vi "FILE Open.vi"(5 "Pattern":string, 6 "Default Name":string, 7 "Dialog Prompt":string, 8 "Error In (no error)":errorcluster, 10 "Start path":path=path "", 11 "File Path (\" \")":path) -> (0 "Error Out":errorcluster, 1 "Size (bytes)":i32, 2 "Dup File Path":path, 3 "Refnum":refnum<file>, 4 "Last Mod":u32)   [LabVIEW 2011]
doc: "This VI opens a file at the file path specified and returns the file's size, mod date, refnum, and dir/file info. If the File Path is empty then a file dialog will appear according to the dialog input parameters given, and the file chosen will be opened. If the file dialog is canceled then execution will continue with no errors.\n\nThis vi was created by David Gianetto, contact me with any problems, questions, etc."
uses:
  Type Defs/FILE Open Mode Enum.ctl
panel:
  out "Directory":bool
  in  "Open Mode (0)":T1
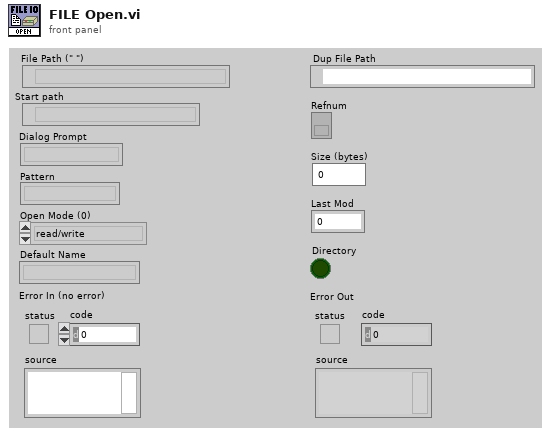
[diagram p1: front panel]
types:
  T1 = typedef "FILE Open Mode Enum.ctl" = enum16{"read/write", "read-only", "write-only", "write-only (truncate)"}
  T2 = enum32{"existing file", "new file", "new or existing file", "existing dir", "new dir", "new or existing dir", "existing file (use LLBs)", "new file (use LLBs)", "new or existing file (use LLBs)", "new or existing file or directory (use LLBs)"}
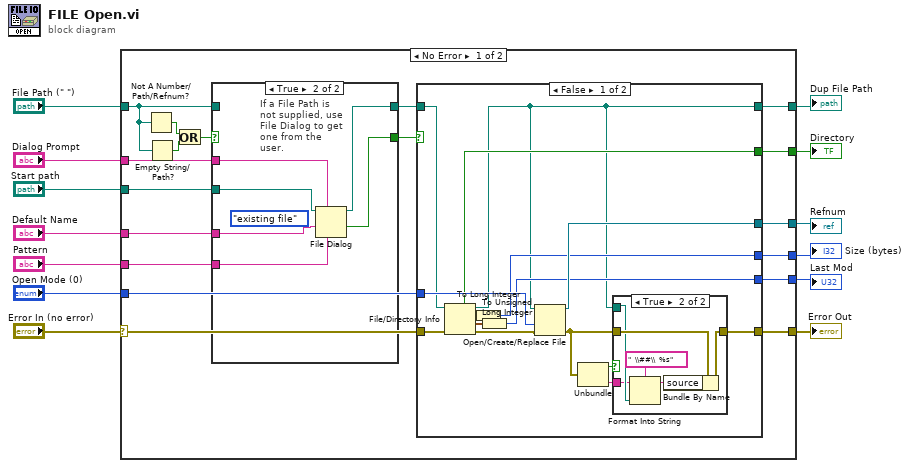
[diagram p0: block diagram]
diagram:
  n1 = case shown="No Error" "Error In (no error)" {
    selector: "Error In (no error)" -> [w14 w63]
    tunnel: [w16 w64] -> w13
    tunnel: [w30 _] -> w7
    tunnel: "File Path (\" \")" -> [w27 w64]
    tunnel: "Dialog Prompt" -> [w26 _]
    tunnel: "Start path" -> [w25 _]
    tunnel: "Default Name" -> [w24 _]
    tunnel: "Pattern" -> [w23 _]
    tunnel: "Open Mode (0)" -> [w22 _]
    tunnel: [w20 _] -> w4
    tunnel: [w19 _] -> w5
    tunnel: [w18 _] -> w3
    tunnel: [w17 w63] -> w2
    frame No Error {
      n2 = Not A Number/Path/Refnum?(number/path/refnum=w27) -> (NaN/Path/Refnum?=w29:bool)
      n3 = Empty String/Path?(string/path=w27) -> (empty?=w28:bool)
      n4 = Or(x=w29, y=w28) -> (x .or. y?=w15:bool)
      n5 = case shown="True" w15 {
        selector: w15 -> [w55 _]
        tunnel: [w55 w62] -> w31
        tunnel: [w56 w61] -> w21
        tunnel: w27 -> [w56 _]
        tunnel: w26 -> [_ w60]
        tunnel: w25 -> [_ w59]
        tunnel: w24 -> [_ w58]
        tunnel: w23 -> [_ w57]
        frame False {
          # "A File Path is supplied (not empty); proceed"
        }
        frame True {
          (unwired) T2."existing file" ("select mode (2)")
          # "If a File Path is not supplied, use File Dialog to get one from the user."
          n6 = File Dialog(6:w57, 7:w60, 9:w58, 11:w59) -> (1:w62:bool, 3:w61:path)  [unwired: 1 in, 4 out]
        }
      }
      n7 = case shown="False" w31 {
        tunnel: w21 -> [w44 _]
        tunnel: [w37 _] -> w16
        tunnel: [w46 _] -> w30
        tunnel: w22 -> [w45 _]
        tunnel: [w35 w54] -> w17
        tunnel: w14 -> [w43 w54]
        tunnel: [w42 _] -> w20
        tunnel: [w41 _] -> w19
        tunnel: [w40 _] -> w18
        frame False {
          n8 = File/Directory Info(path=w44, error in=w43) -> (path out=w37:path, directory=w42:bool, size=w32:i64, last mod=w39:timestamp, error out=w33:errorcluster)  [unwired: 2 out]
          n9 = To Long Integer(number=w32) -> (32bit integer=w41:i32)
          n10 = To Unsigned Long Integer(number=w39) -> (unsigned 32bit integer=w40:u32)
          n11 = Open/Create/Replace File(file path (use dialog)=w37, error in=w33, access (0:read/write)=w45) -> (refnum out=w46:refnum<file>, error out=w36:errorcluster)  [unwired: 4 out]
          n12 = Unbundle(w36) -> ("status"=w38:bool, "source"=w34:string)  [unwired: 1 out]
          n13 = case shown="True" w38 {
            tunnel: [w47 w51] -> w35
            tunnel: w36 -> [w47 w50]
            tunnel: w37 -> [_ w49]
            tunnel: w34 -> [_ w48]
            frame False {
            }
            frame True {
              n14 = Format Into String(format string="  \\##\\  %s", initial string=w48, w49) -> (resulting string=w52:string)  [unwired: 1 in, 1 out]
              n15 = Bundle By Name(cluster=w50, "source"=w52) -> (w51:errorcluster)
            }
          }
        }
        frame True {
          # "Cancelled"
        }
      }
    }
    frame Error {
    }
  }
  "Dup File Path" <- w13
  "Refnum" <- w7
  "Error Out" <- w2
  "Size (bytes)" <- w5
  "Directory" <- w4
  "Last Mod" <- w3
